vi "Initialize Data Buffer.vi"(11 "Output Groups":T1[](array[typedef])) -> (3 "Data Buffers":cluster{"Data":dbl[]}[](array[cluster]))   [LabVIEW 2021, in "Modbus Master Engine.lvlib"]
uses:
  Modbus Master Engine.lvlib
  Bulk Data Access.ctl
  System Explorer/SubVIs/Modbus Type.ctl
  Shared/Controls/Data Model/Channel.ctl
  <vilib>/NI VeriStand/Custom Device API/Custom Device Channel Type.ctl
  Shared/Controls/Data Model/Mapping.ctl
  Shared/Controls/Data Model/DataType.ctl
  <vilib>/NI VeriStand/Custom Device API/Custom Device Item Ref.ctl
  Shared/Modbus Master Shared.lvlib
  <vilib>/NI VeriStand/Custom Device API/Custom Device API.lvlib
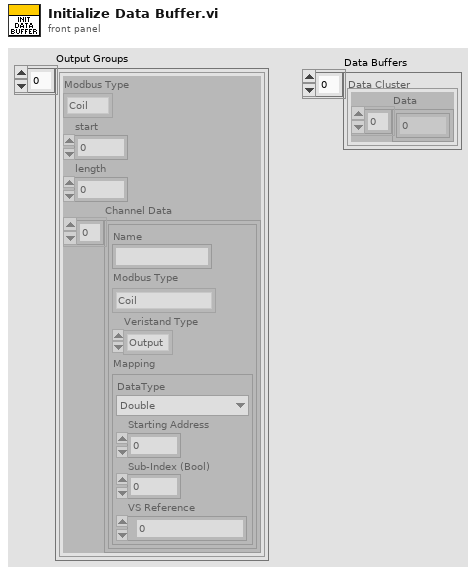
[diagram p1: front panel]
types:
  T1 = typedef "Modbus Master Shared.lvlib/Bulk Data Access.ctl" = cluster{"Modbus Type":T2, "start":u16, "length":u16, "Channel Data":T3[]}
  T2 = typedef "Modbus Master Shared.lvlib/Modbus Type.ctl" = enum16{"Coil", "Discrete Input", "Holding Register", "Input Register"}
  T3 = typedef "Modbus Master Shared.lvlib/Channel.ctl" = cluster{"Name":string, "Modbus Type":T2, "Veristand Type":T4, "Mapping":T5}
  T4 = typedef "Custom Device API.lvlib/Custom Device Channel Type.ctl" = enum16{"Input", "Output"}
  T5 = typedef "Modbus Master Shared.lvlib/Mapping.ctl" = cluster{"DataType":T6, "Starting Address":u16, "Sub-Index (Bool)":u16, "VS Reference":T7}
  T6 = typedef "Modbus Master Shared.lvlib/DataType.ctl" = enum16{"Double", "Single", "I64", "I32", "I16", "I8", "U64", "U32", "U16", "U8", "Boolean"}
  T7 = typedef "Custom Device API.lvlib/Custom Device Item Ref.ctl" = u64
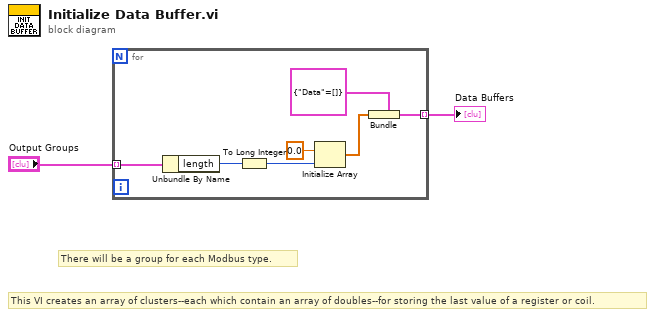
[diagram p0: block diagram]
diagram:
  # "There will be a group for each Modbus type."
  # "This VI creates an array of clusters--each which contain an array of doubles--for storing the last value of a register or coil."
  n1 = for {
    tunnel: [w9] -> w2 mode=indexing
    tunnel: "Output Groups" -> [w7] mode=indexing
    n2 = Unbundle By Name(w7) -> ("length"=w4:u16)
    n3 = To Long Integer(number=w4) -> (32bit integer=w3:i32)
    n4 = Initialize Array(0.0 ("element"), w3) -> (w5:dbl[])
    n5 = Bundle(cluster=cluster{"Data":dbl[]} {"Data"=[]}, "Data"=w5) -> (w9:cluster{"Data":dbl[]})
  }
  "Data Buffers" <- w2
